vi "ScopeInstruments_CallCreateSessionsWithUnregisteredSessionsReserved_RemoteSessionsCreated.vi"(8 "error in":errorcluster) -> (0 "error out":errorcluster, 2 "result":string, 3 "pass":bool)   [LabVIEW 2020, in "MeasurementServerTests.lvlib"]
uses:
  MeasurementServerTests.lvlib
  Runtime/MeasurementLink niScope/MeasurementLink niScope.lvlib
  Runtime/MeasurementLink niScope/Create Sessions - NSess.vi
  c4a911aa-80ea-4246-aa9a-6d8f5dfeb207.vi
  Runtime/MeasurementLink Session Management/Session Reservation/Session Reservation.lvclass
panel:
  out "session reservation out":refnum<class "Session Reservation.lvclass">
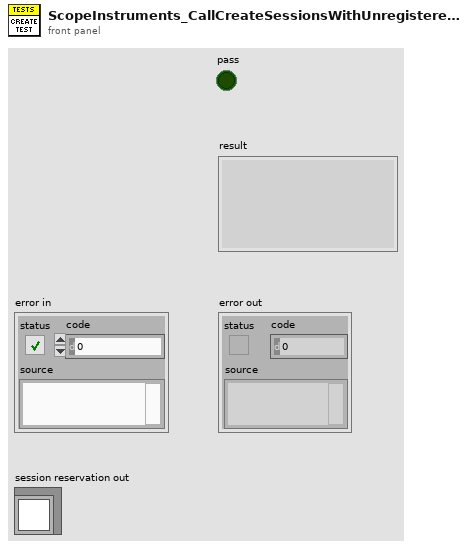
[diagram p1: front panel]
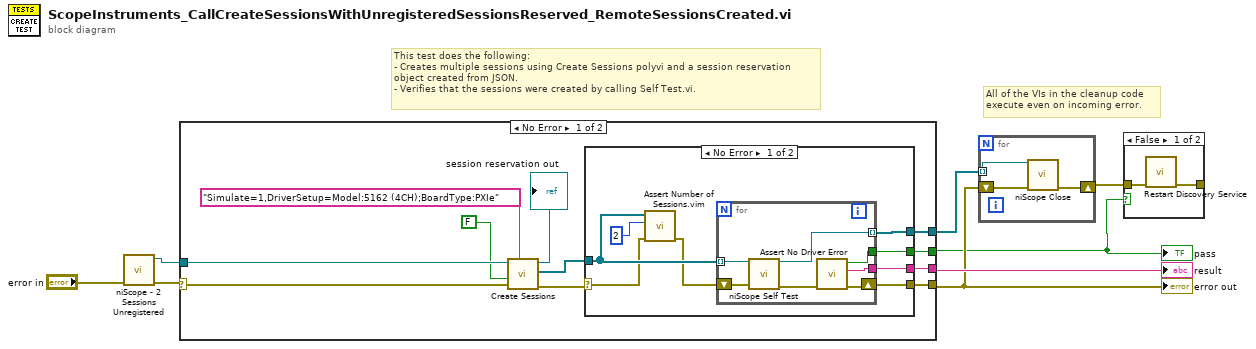
[diagram p0: block diagram]
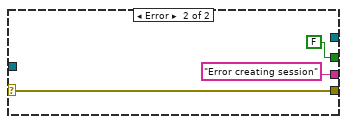
[diagram p2: hidden frame]
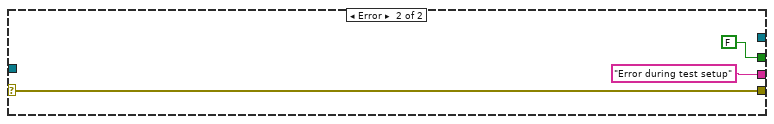
[diagram p3: hidden frame]
diagram:
  # "All of the VIs in the cleanup code\nexecute even on incoming error."
  # "This test does the following:\n- Creates multiple sessions using Create Sessions polyvi and a session reservation\nobject created from JSON.\n- Verifies that the sessions were created by calling Self Test.vi."
  n1 = call "niScope - 2 Sessions Unregistered.vi"("error in"="error in") -> ("error out"=w4:errorcluster, "Session Reservation out"=w3:refnum<class "Session Reservation.lvclass">)  [unwired: 9 in]
  n2 = case shown="No Error" w4 {
    selector: w4 -> [w12 w38]
    tunnel: [w18 w38] -> w6
    tunnel: [w19 FALSE] -> w1
    tunnel: [w17 "Error during test setup" ("f")] -> w8
    tunnel: [w16 _] -> w7
    tunnel: w3 -> [w11 _]
    frame No Error {
      n3 = call-poly "Create Sessions.vi"("option string"="Simulate=1,DriverSetup=Model:5162 (4CH);BoardType:PXIe", "error in"=w12, "reset"=FALSE, "session reservation in"=w11) -> ("error out"=w10:errorcluster, "sessions"=w13:refnum<k15>[], "session reservation out"=→"session reservation out":refnum<class "Session Reservation.lvclass">)  [unwired: 4 in, 1 out]
      n4 = case shown="No Error" w10 {
        selector: w10 -> [w21 w36]
        tunnel: [w27 FALSE] -> w19
        tunnel: [w25 w36] -> w18
        tunnel: [w26 "Error creating session"] -> w17
        tunnel: w13 -> [w23 _]
        tunnel: [w24 _] -> w16
        frame No Error {
          n5 = call "Assert Number of Sessions.vim"("error in"=w21, "expected number of sessions"=2, "sessions"=w23) -> ("error out"=w22:errorcluster)  [unwired: 6 in, 2 out]
          n6 = for {
            tunnel: [w34] -> w27
            tunnel: [w33] -> w26
            tunnel: [w31] -> w24 mode=indexing
            tunnel: w23 -> [w29] mode=indexing
            shift-right: [w32] -> w25
            shift-left: w22 -> [w28]
            n7 = call <instrlib>:"niScope Self Test.vi"("instrument handle"=w29, "error in"=w28) -> ("instrument handle out"=w31:refnum<k15>, "error out"=w30:errorcluster)  [unwired: 10 in, 2 out]
            n8 = call "Assert No Driver Error.vi"("error in"=w30) -> ("error out"=w32:errorcluster, "result"=w33:string, "pass?"=w34:bool)  [unwired: 8 in]
          }
        }
        frame Error {
        }
      }
    }
    frame Error {
    }
  }
  "error out" <- w6
  "pass" <- w1
  "result" <- w8
  n9 = for {
    tunnel: w7 -> [w43] mode=indexing
    shift-right: [w42] -> w2
    shift-left: w6 -> [w41]
    n10 = call <instrlib>:"niScope Close.vi"("instrument handle"=w43, "error in"=w41) -> ("error out"=w42:errorcluster)  [unwired: 13 in]
  }
  n11 = case shown="False" w1 {
    tunnel: w2 -> [w45 _]
    tunnel: [w44 _] -> _
    frame False {
      n12 = call "Restart Discovery Service.vi"("error in"=w45) -> ("error out"=w44:errorcluster)  [unwired: 10 in]
    }
    frame True {
    }
  }
